vi "FPGA (Top Level).vi"() -> ()   [LabVIEW 2017]
uses:
  <vilib>/LabVIEW Targets/FPGA/cRIO/cRIO-9505/controls.llb/_nicrio_cRIO-9505_DriveStatus.ctl
  <vilib>/Platform/TimedLoop/XDataNode/timing_clust.ctl
  <vilib>/Platform/TimedLoop/XDataNode/nitl_modes.ctl
  <vilib>/Platform/TimedLoop/XDataNode/wakeup.ctl
  <vilib>/rvi/FXPMathLib/FxpSinAndCos/subVIs/nifxpmath_SinAndCos_SimConfig.ctl
  <vilib>/rvi/Emulation/niFpgaGetClockAttributes.vi
  <vilib>/rvi/Emulation/niFpgaSctlEmulationGetInTimedLoop.vi
  <vilib>/rvi/Emulation/niFpgaEmulationReportErrorSimple.vi
  <vilib>/rvi/eio/common/nirviEmuTemplateMethod_errors.vi
  <vilib>/rvi/Emulation/niFpgaEmulationIsFPGAContextNoSignature.vi
  <vilib>/rvi/DataTransferAndStorage/Container/Common/niFpgaContainerGetUniqueNameForEmu.vi
  <vilib>/rvi/Memory/Memory_Emulation/niFpgaMemoryEmulationCacheClearOnFirstRun.vi
  <vilib>/rvi/Memory/Memory_Emulation/nirvimemoryEmulationManagerCache_MakeExclusive.vi
  <vilib>/rvi/Memory/Memory_Emulation/niFpgaMemoryEmulationValidateCache.vi
  <vilib>/rvi/Memory/Memory_Emulation/nirvimemoryEmulationManagerCache_InsertValue.vi
  <vilib>/Utility/error.llb/Clear Errors.vi
  <vilib>/rvi/Memory/Memory_Emulation/nirvimemoryEmulationManagerCache_ReleaseExclusive.vi
  <vilib>/rvi/Memory/Memory_Emulation/nirvimemoryEmulationManagerCache_GetValue.vi
  <vilib>/rvi/Memory/Memory_Emulation/nirvimemoryEmulationManagerCache_SetValue.vi
  <vilib>/rvi/Emulation/niFpgaProcessEmulError.vi
  <vilib>/rvi/Emulation/niFpgaCriticalErrorInLSC.vi
  <vilib>/rvi/FXPMathLib/FxpSinAndCos/simVIs/DllFxpSinAndCosTemp_sub.vi
  <vilib>/eio/EIONode/EIONode.xnode
  <vilib>/rvi/DataTransferAndStorage/Container/XNode/niFpgaContainer.xnode
  <vilib>/rvi/DataTransferAndStorage/Register/Emulation/niFpgaRegisterEmulation.vi
  <vilib>/rvi/FXPMathLib/FxpSinAndCos/XNode/nifxpmath_SinAndCos.xnode
  <vilib>/Platform/TimedLoop/XDataNode/XDataNode.xnode
  <vilib>/Platform/TimedLoop/XDataNode/XDNodeRunTimeDep.lvlib
  <vilib>/eio/EIOMethodNode/EIOMethodNode.xnode
panel:
  out "x .or. y?":u8
  out "PWM Period (ticks)":u32
  out "Link 2 PWM Duty (Counts)":i32
  out "Link 1 PWM Duty (Counts)":i32
  in  "PWM Gen Period (ms)":u16=10
  in  "Enable Output V":bool
  in  "PWM Period Loops":i32=200
  in  "Link_1 Duty":fxp<+/-,32,0>
  in  "Link_2 Duty":fxp<+/-,32,0>
  in  "LINK1_DRIVE_ENABLED":bool
  in  "LINK2_DRIVE_ENABLED":bool
  out "LINK2_DRIVE_STATUS":T1
  out "LINK1_DRIVE_STATUS":T1
  in  "LINK1_LENGTH_MM":fxp<+,16,12>=2.0 format="%#_19g"
  in  "LINK2_LENGTH_MM":fxp<+,16,12>=2.0 format="%#_19g"
  in  "X_OFFSET_MM":fxp<+/-,33,15>
  in  "Y_OFFSET_MM":fxp<+/-,33,15>
  out "LINK2_Y_MM":fxp<+/-,34,16>
  out "LINK2_X_MM":fxp<+/-,34,16>
  out "LINK1_Y_MM":fxp<+/-,34,16>
  out "LINK1_X_MM":fxp<+/-,34,16>
  out "LINK1_ENC_POS":i32
  out "LINK2_ENC_POS":i32
  out "LINK1_POT_POS":i32
  out "LINK2_POT_POS":i32
  in  "LINK1_ENC_SCALE":fxp<+,32,0> format="%#_32g"
  in  "LINK2_ENC_SCALE":fxp<+,32,0>=0.029296900611370802 format="%#_32g"
  in  "LINK1_PWM_MAX":i16
  in  "LINK2_PWM_MAX":i16
  in  "LINK1_DEMAND_PWM":i16
  in  "LINK2_DEMAND_PWM":i16
  in  "LINK1_POT_SCALE":fxp<+/-,32,16>
  in  "LINK1_OFFSET":fxp<+/-,16,16>
  in  "LINK2_POT_SCALE":fxp<+/-,32,16>
  in  "LINK2_OFFSET":fxp<+/-,16,16>
  in  "AI_POT_LOOP_US":u16=10
  in  "ENC_DEBOUNCE_CYCLES":u16=5
  in  "LINK1_ENC_CNTS":i32
  in  "LINK2_ENC_CNTS":i32
  in  "LINK1_UPDATE_ENC":bool
  in  "LINK2_UPDATE_ENC":bool
  # "PWM at 50kHz"
  # "10MHz Loops Rate"
  # "3.3V"
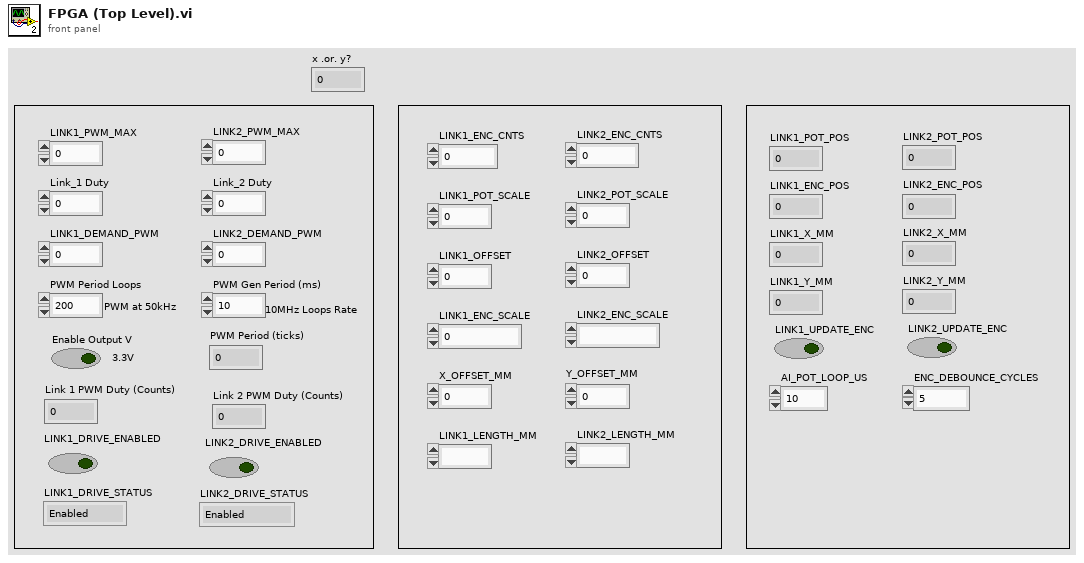
[diagram p1: front panel]
types:
  T1 = typedef "_nicrio_cRIO-9505_DriveStatus.ctl" = enum8{"Enabled", "Disabled", "Disabled by Drive Fault", "Disabled by Temp. Fault", "Disabled by E-Stop", "Unknown"}
  T2 = typedef "XDNodeRunTimeDep.lvlib/timing_clust.ctl" = cluster{"Expected End [f-1]":u64, "Actual End [f-1]":u64, "Finished Late? [f-1]":bool, "Expected End [i-1]":u64, "Actual End [i-1]":u64, "Finished Late? [i-1]":bool, "Expected Start [i]":u64, "Actual Start [i]":u64, "Expected Start [f]":u64, "Actual Start [f]":u64, "Source Name":string, "Structure Name":string, "Period":i64, "Deadline":i64, "Offset":i64, "Start":i64, "Priority":i32, "Timeout":i32, "Mode":T3, "Wakeup Reason":T4, "Error":errorcluster, "Source Type":string, "Secondary Source Type":string, "Global End Time":u64, "Global Start Time":u64, "Frame Duration":u64, "Iteration Duration":u64, "Assigned CPU":i32, "I/O Scan Engine Mode":u32}
  T3 = typedef "XDNodeRunTimeDep.lvlib/nitl_modes.ctl" = enum32{"No Change", "Process missed periods, maintain original phase", "Discard missed periods, maintain original phase", "Process missed periods, ignore original phase", "Discard missed periods, ignore original phase"}
  T4 = typedef "XDNodeRunTimeDep.lvlib/wakeup.ctl" = enum32{"Normal", "Aborted", "Asynchronous wakeup", "Timing source error", "Timed loop error", "Timeout"}
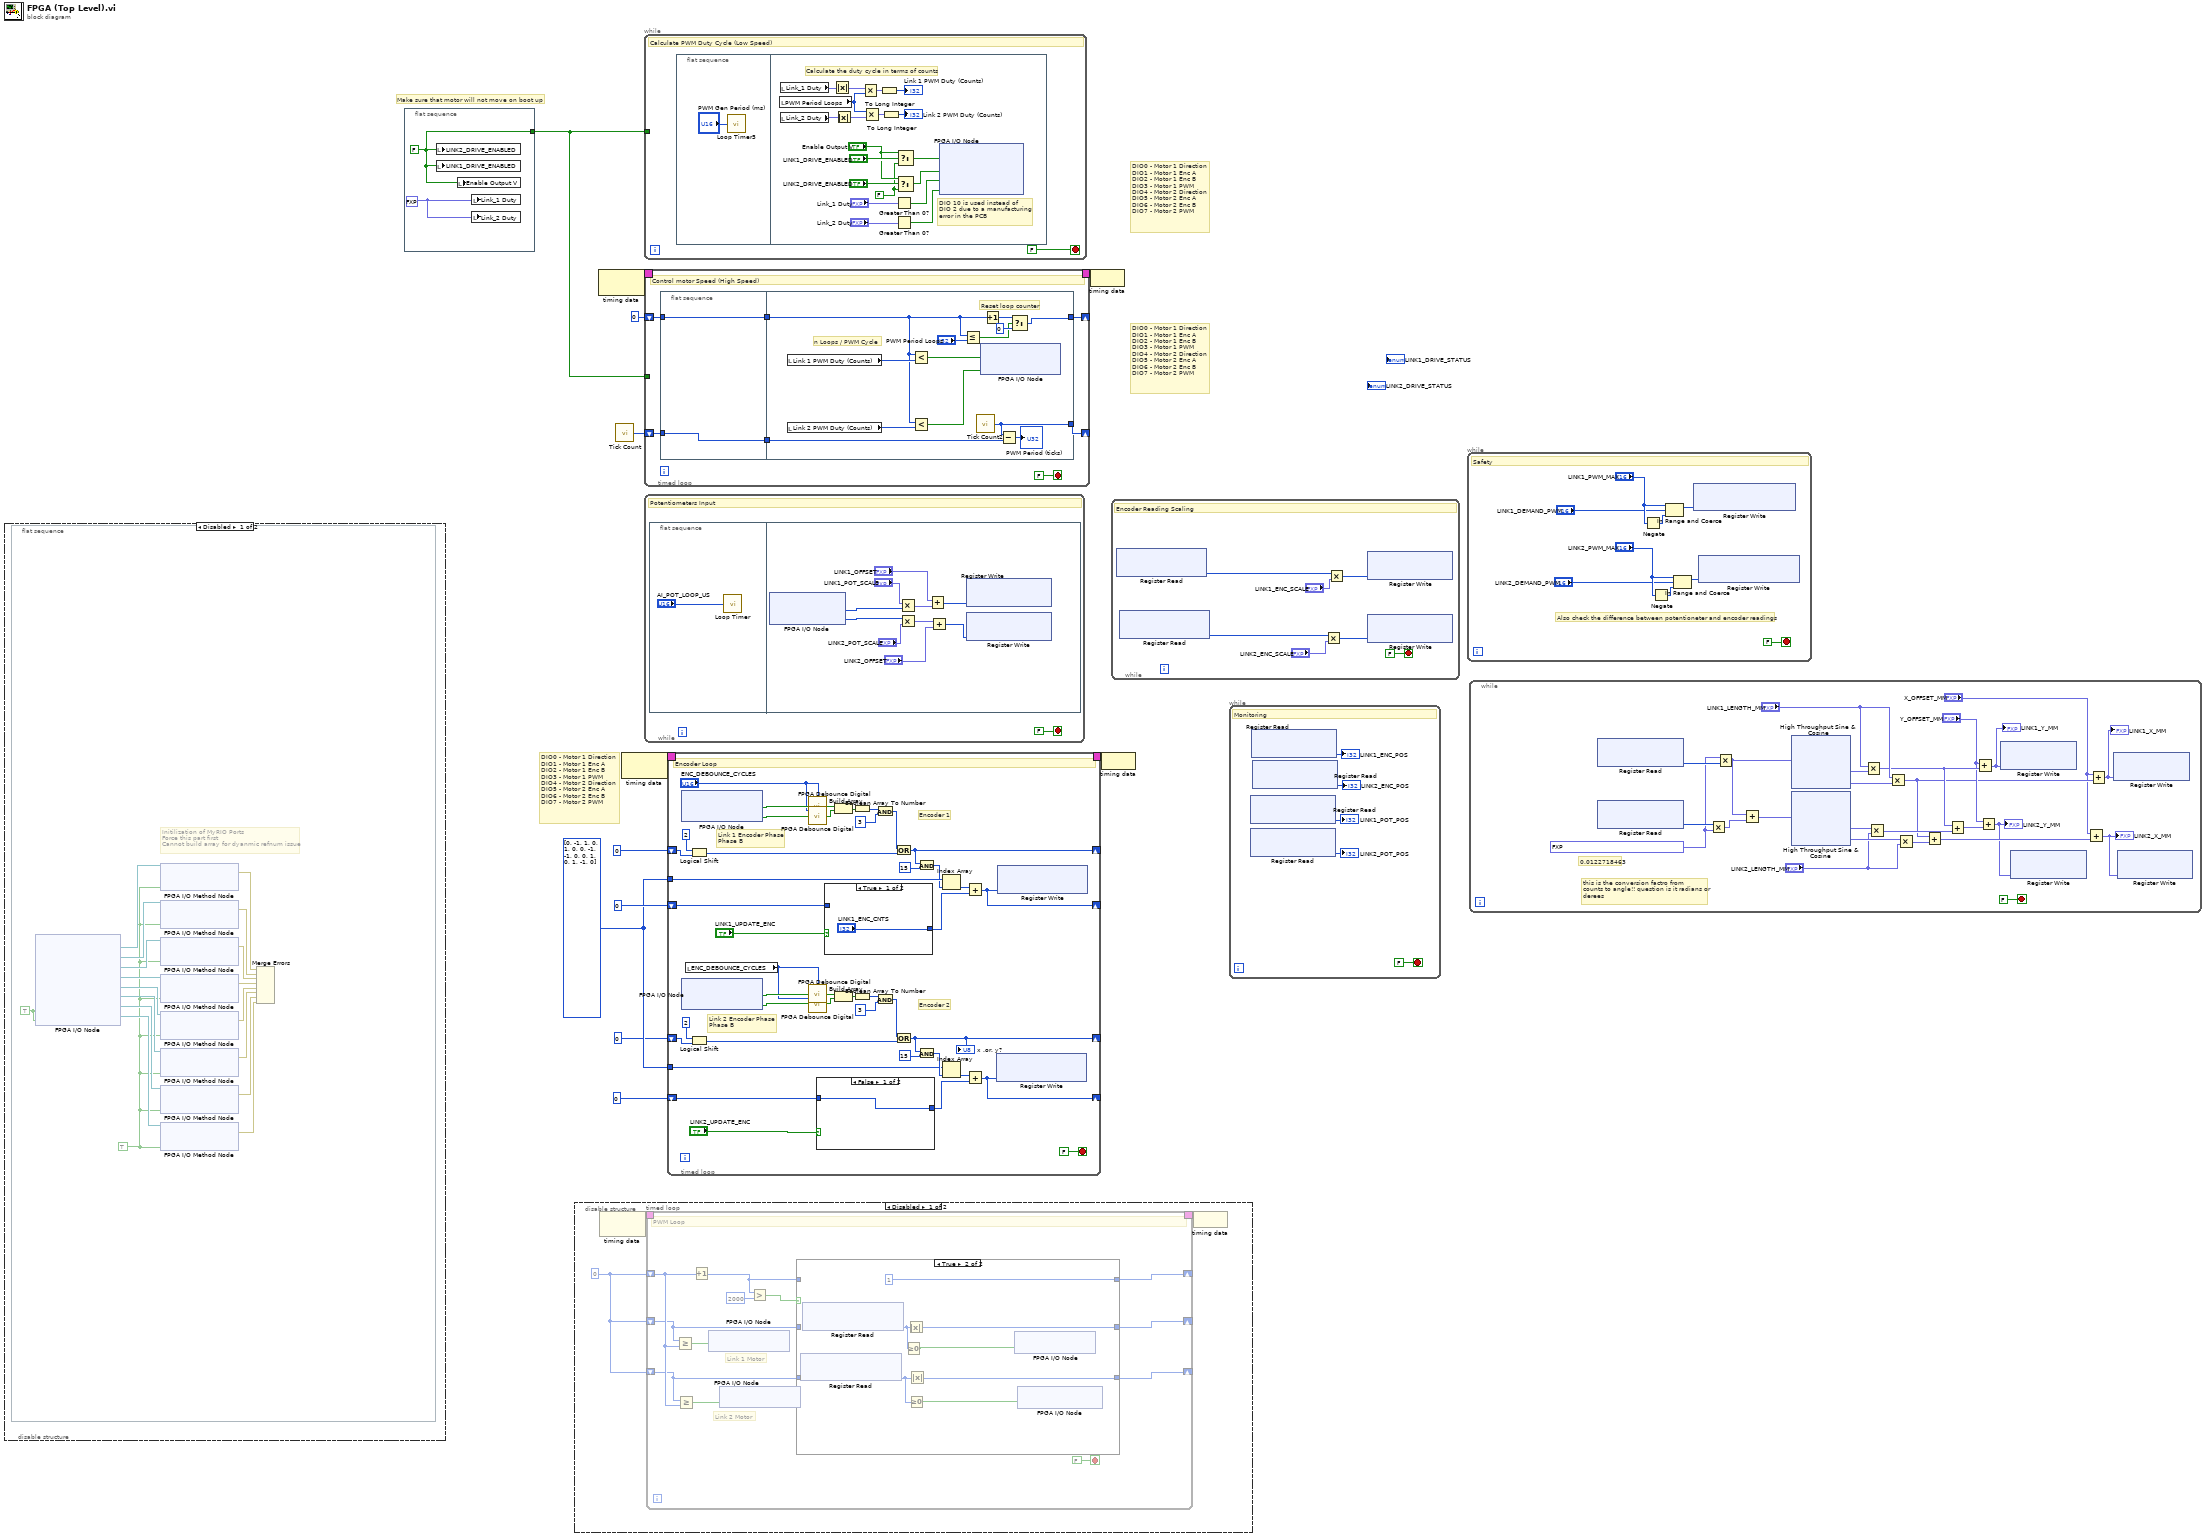
[diagram p0: block diagram]
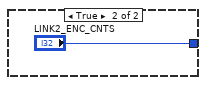
[diagram p5: hidden frame]
diagram:
  w8 = i8[] [0, -1, 1, 0, 1, 0, 0, -1, -1, 0, 0, 1, 0, 1, -1, 0]
  # "DIO0 - Motor 1 Direction \nDIO1 - Motor 1 Enc A\nDIO2 - Motor 1 Enc B\nDIO3 - Motor 1 PWM\nDIO4 - Motor 2 Direction\nDIO5 - Motor 2 Enc A\nDIO6 - Motor 2 Enc B\nDIO7 - Motor 2 PWM"
  # "DIO0 - Motor 1 Direction \nDIO1 - Motor 1 Enc A\nDIO2 - Motor 1 Enc B\nDIO3 - Motor 1 PWM\nDIO4 - Motor 2 Direction\nDIO5 - Motor 2 Enc A\nDIO6 - Motor 2 Enc B\nDIO7 - Motor 2 PWM"
  # "DIO0 - Motor 1 Direction \nDIO1 - Motor 1 Enc A\nDIO2 - Motor 1 Enc B\nDIO3 - Motor 1 PWM\nDIO4 - Motor 2 Direction\nDIO5 - Motor 2 Enc A\nDIO6 - Motor 2 Enc B\nDIO7 - Motor 2 PWM"
  # "Make sure that motor will not move on boot up"
  n1 = disable-structure shown="Disabled" {
    frame Disabled {
      n2 = flat-sequence {
        frame #0 {
          w21 = TRUE ("Link 2 Encoder Phase B")
          w30 = TRUE ("Link 2 Encoder Phase B")
          # "Initilization of MyRIO Ports\nForce this part first \nCannot build array for dyanmic refnum issue"
          n3 = xnode "FPGA I/O Node"("ConnectorA/DIO5"=w30, "ConnectorA/DIO10"=w30) -> ("FPGA I/O Out"=w29:refnum<k21>, "FPGA I/O Out"=w28:refnum<k21>, "FPGA I/O Out"=w27:refnum<k21>, "FPGA I/O Out"=w26:refnum<k21>, "FPGA I/O Out"=w25:refnum<k21>, "FPGA I/O Out"=w24:refnum<k21>, "FPGA I/O Out"=w23:refnum<k21>, "FPGA I/O Out"=w22:refnum<k21>)  [unwired: 8 in, 6 out]
          n4 = xnode "FPGA I/O Method Node"("FPGA I/O In"=w29, "Enable"=w21) -> ("error out"=w20:errorcluster)  [unwired: 1 in, 1 out]
          n5 = xnode "FPGA I/O Method Node"("FPGA I/O In"=w28, "Enable"=w21) -> ("error out"=w19:errorcluster)  [unwired: 1 in, 1 out]
          n6 = xnode "FPGA I/O Method Node"("FPGA I/O In"=w27, "Enable"=w21) -> ("error out"=w18:errorcluster)  [unwired: 1 in, 1 out]
          n7 = xnode "FPGA I/O Method Node"("FPGA I/O In"=w26, "Enable"=w21) -> ("error out"=w17:errorcluster)  [unwired: 1 in, 1 out]
          n8 = xnode "FPGA I/O Method Node"("FPGA I/O In"=w25, "Enable"=w21) -> ("error out"=w16:errorcluster)  [unwired: 1 in, 1 out]
          n9 = xnode "FPGA I/O Method Node"("FPGA I/O In"=w24, "Enable"=w21) -> ("error out"=w15:errorcluster)  [unwired: 1 in, 1 out]
          n10 = xnode "FPGA I/O Method Node"("FPGA I/O In"=w23, "Enable"=w21) -> ("error out"=w14:errorcluster)  [unwired: 1 in, 1 out]
          n11 = xnode "FPGA I/O Method Node"("FPGA I/O In"=w22, "Enable"=w21) -> ("error out"=w13:errorcluster)  [unwired: 1 in, 1 out]
          n12 = Merge Errors(w20, w19, w18, w17, w16, w15, w14, w13) -> ()  [unwired: 1 out]
        }
      }
    }
    frame Enabled {
    }
  }
  n13 = flat-sequence {
    tunnel: [w31] -> w1
    frame #0 {
      w32 = fxp<+/-,32,0> 0.0 ("Link_1 Duty")
      w31 = FALSE ("LINK2_DRIVE_ENABLED")
      n14 = local write "LINK2_DRIVE_ENABLED"(w31) -> ()
      n15 = local write "LINK1_DRIVE_ENABLED"(w31) -> ()
      n16 = local write "Enable Output V"(w31) -> ()
      n17 = local write "Link_1 Duty"(w32) -> ()
      n18 = local write "Link_2 Duty"(w32) -> ()
    }
  }
  n19 = disable-structure shown="Disabled" {
    frame Disabled {
      w33 = i16 0 ("Motor 1 PWM Duty Cycle")
      n20 = node-c288() -> (w35:T2)  [unwired: 1 in]
      n21 = timed-loop {
        timing: w35 -> [_]
        timing-out: [_] -> w34
        shift-right: [w46] -> _
        shift-left: w33 -> [w45]
        shift-right: [w44] -> _
        shift-left: w33 -> [w42]
        shift-right: [w43] -> _
        shift-left: w33 -> [w41]
        stop <- FALSE stop-if-true
        # "Link 2 Motor"
        # "Link 1 Motor"
        # "PWM Loop"
        n22 = Greater Or Equal?(x=w42, y=w45) -> (x >= y?=w37:bool)
        n23 = Greater Or Equal?(x=w41, y=w45) -> (x >= y?=w36:bool)
        n24 = Increment(x=w45) -> (x+1=w39:i16)
        n25 = xnode "FPGA I/O Node"("ConnectorA/DIO8"=w37) -> ()  [unwired: 1 in, 1 out]
        n26 = xnode "FPGA I/O Node"("ConnectorA/DIO9"=w36) -> ()  [unwired: 1 in, 1 out]
        n27 = Greater?(x=w39, y=i16 2000) -> (0:w40:bool)
        n28 = case shown="True" w40 {
          tunnel: w39 -> [w50 _]
          tunnel: [w50 i16 1 ("Motor 1 PWM Duty Cycle")] -> w46
          tunnel: [w49 w56] -> w44
          tunnel: [w48 w55] -> w43
          tunnel: w42 -> [w49 _]
          tunnel: w41 -> [w48 _]
          frame False {
          }
          frame True {
            n29 = xnode ("Register Read")() -> ("Data"=w53:i16)  [unwired: 1 in, 1 out]
            n30 = xnode ("Register Read")() -> ("Data"=w54:i16)  [unwired: 1 in, 1 out]
            n31 = Greater Or Equal To 0?(x=w54) -> (x >= 0?=w51:bool)
            n32 = Absolute Value(x=w54) -> (abs(x)=w56:i16)
            n33 = Greater Or Equal To 0?(x=w53) -> (x >= 0?=w52:bool)
            n34 = Absolute Value(x=w53) -> (abs(x)=w55:i16)
            n35 = xnode "FPGA I/O Node"("ConnectorA/DIO6"=w51) -> ()  [unwired: 1 in, 1 out]
            n36 = xnode "FPGA I/O Node"("ConnectorA/DIO10"=w52) -> ()  [unwired: 1 in, 1 out]
          }
        }
      }
      n37 = node-c288(w34) -> ()
    }
    frame Enabled {
    }
  }
  n38 = node-c288() -> (w4:T2)  [unwired: 1 in]
  n39 = call "Tick Count"() -> ("Tick Count(Ticks)"=w5:u32)
  n40 = node-c288() -> (w12:T2)  [unwired: 1 in]
  n41 = while {
    tunnel: w1 -> [_]
    stop <- FALSE stop-if-true
    # "Calculate PWM Duty Cycle (Low Speed)"
    n42 = flat-sequence {
      frame #0 {
        n43 = call "Loop Timer3"("Count(mSec)"="PWM Gen Period (ms)") -> ()  [unwired: 1 out]
      }
      frame #1 {
        w70 = FALSE
        # "DIO 10 is used instead of \nDIO 2 due to a manufacturing \nerror in the PCB"
        # "Calculate the duty cycle in terms of counts"
        n44 = local read "PWM Period Loops"() -> (w74:i32)
        n45 = local read "Link_1 Duty"() -> (w79:fxp<+/-,32,0>)
        n46 = local read "Link_2 Duty"() -> (w75:fxp<+/-,32,0>)
        n47 = Absolute Value(x=w79) -> (abs(x)=w80:fxp<+,32,0>)
        n48 = Absolute Value(x=w75) -> (abs(x)=w76:fxp<+,32,0>)
        n49 = Multiply(x=w80, y=w74) -> (x*y=w81:fxp<+/-,63,31>)
        n50 = Multiply(x=w74, y=w76) -> (x*y=w78:fxp<+/-,63,31>)
        n51 = To Long Integer(number=w81) -> (32bit integer=→"Link 1 PWM Duty (Counts)":i32)
        n52 = To Long Integer(number=w78) -> (32bit integer=→"Link 2 PWM Duty (Counts)":i32)
        n53 = Greater Than 0?(x="Link_1 Duty") -> (x > 0?=w65:bool)
        n54 = Greater Than 0?(x="Link_2 Duty") -> (x > 0?=w64:bool)
        n55 = Select(t="Enable Output V", s="LINK1_DRIVE_ENABLED", f=w70) -> (s? t:f=w69:bool)
        n56 = Select(t="Enable Output V", s="LINK2_DRIVE_ENABLED", f=w70) -> (s? t:f=w68:bool)
        n57 = xnode "FPGA I/O Node"("ConnectorA/DIO10"=w69, "ConnectorA/DIO7"=w68, "ConnectorA/DIO0"=w65, "ConnectorA/DIO5"=w64) -> ()  [unwired: 4 in, 4 out]
      }
    }
  }
  n58 = timed-loop {
    shift-right: [w88] -> _
    shift-left: w5 -> [w87]
    timing: w4 -> [_]
    timing-out: [_] -> w3
    shift-right: [w85] -> _
    shift-left: i16 0 -> [w84]
    tunnel: w1 -> [_]
    stop <- FALSE stop-if-true
    # "Control motor Speed (High Speed)"
    n59 = flat-sequence {
      tunnel: w87 -> [w91]
      tunnel: [w91] -> w86
      tunnel: w84 -> [w90]
      tunnel: [w90] -> w83
      tunnel: [w100] -> w88
      tunnel: w86 -> [w99]
      tunnel: [w96] -> w85
      tunnel: w83 -> [w93]
      frame #0 {
      }
      frame #1 {
        # "Reset loop counter"
        # "n Loops / PWM Cycle"
        n60 = local read "Link 1 PWM Duty (Counts)"() -> (w102:i32)
        n61 = local read "Link 2 PWM Duty (Counts)"() -> (w101:i32)
        n62 = Less?(x=w93, y=w102) -> (x < y?=w104:bool)
        n63 = Less?(x=w93, y=w101) -> (x < y?=w103:bool)
        n64 = Less Or Equal?(x=w93, y="PWM Period Loops") -> (x <= y?=w92:bool)
        n65 = call "Tick Count2"() -> ("Tick Count(Ticks)"=w100:u32)
        n66 = xnode "FPGA I/O Node"("ConnectorA/DIO1"=w104, "ConnectorA/DIO6"=w103) -> ()  [unwired: 2 in, 2 out]
        n67 = Increment(x=w93) -> (x+1=w97:i16)
        n68 = Subtract(x=w100, y=w99) -> (x-y=→"PWM Period (ticks)":u32)
        n69 = Select(t=w97, s=w92, f=i16 0) -> (s? t:f=w96:i16)
      }
    }
  }
  n70 = while {
    stop <- FALSE stop-if-true
    # "Potentiometers Input"
    n71 = flat-sequence {
      frame #0 {
        n72 = call "Loop Timer"("Count(uSec)"="AI_POT_LOOP_US") -> ()  [unwired: 1 out]
      }
      frame #1 {
        n73 = xnode "FPGA I/O Node"() -> ("ConnectorA/AI1"=w110:u16, "ConnectorA/AI2"=w109:u16)  [unwired: 2 in, 2 out]
        n74 = Multiply(x="LINK1_POT_SCALE", y=w110) -> (x*y=w117:fxp<+/-,48,32>)
        n75 = Multiply(x=w109, y="LINK2_POT_SCALE") -> (x*y=w113:fxp<+/-,48,32>)
        n76 = Add(x="LINK1_OFFSET", y=w117) -> (x+y=w111:i32)
        n77 = Add(x=w113, y="LINK2_OFFSET") -> (x+y=w112:i32)
        n78 = xnode ("Register Write")("Data"=w111) -> ()  [unwired: 1 in, 1 out]
        n79 = xnode ("Register Write")("Data"=w112) -> ()  [unwired: 1 in, 1 out]
      }
    }
  }
  n80 = timed-loop {
    timing: w12 -> [_]
    timing-out: [_] -> w11
    tunnel: w8 -> [w158]
    shift-right: [w151] -> _
    shift-left: u8 0 -> [w160]
    shift-right: [w122] -> _
    shift-left: 0 -> [w143]
    tunnel: w8 -> [w127]
    shift-right: [w125] -> _
    shift-left: u8 0 -> [w126]
    shift-right: [w121] -> _
    shift-left: 0 -> [w119]
    stop <- FALSE stop-if-true
    # "Link 2 Encoder Phase \nPhase B"
    # "Link 1 Encoder Phase \nPhase B"
    # "Encoder 2"
    # "Encoder 1"
    # "Encoder Loop"
    n81 = xnode "FPGA I/O Node"() -> ("ConnectorA/DIO4"=w149:bool, "ConnectorA/DIO3"=w148:bool)  [unwired: 2 in, 2 out]
    n82 = xnode "FPGA I/O Node"() -> ("ConnectorA/DIO9"=w133:bool, "ConnectorA/DIO8"=w132:bool)  [unwired: 2 in, 2 out]
    n83 = local read "ENC_DEBOUNCE_CYCLES"() -> (w124:u16)
    n84 = Logical Shift(y=i16 2, x=w160) -> (x << y=w153:u8)
    n85 = Logical Shift(y=i16 2, x=w126) -> (x << y=w136:u8)
    n86 = call "FPGA Debounce Digital.vi"("Input Signal"=w149, "Cycles to Filter"="ENC_DEBOUNCE_CYCLES") -> ("Output Filtered Signal"=w147:bool)
    n87 = call "FPGA Debounce Digital.vi"("Input Signal"=w148, "Cycles to Filter"="ENC_DEBOUNCE_CYCLES") -> ("Output Filtered Signal"=w146:bool)
    n88 = call "FPGA Debounce Digital.vi"("Input Signal"=w133, "Cycles to Filter"=w124) -> ("Output Filtered Signal"=w131:bool)
    n89 = call "FPGA Debounce Digital.vi"("Input Signal"=w132, "Cycles to Filter"=w124) -> ("Output Filtered Signal"=w130:bool)
    n90 = case shown="False" "LINK2_UPDATE_ENC" {
      tunnel: w119 -> [w162 _]
      tunnel: [w162 "LINK2_ENC_CNTS"] -> w128
      frame False {
      }
      frame True {
      }
    }
    n91 = case shown="True" "LINK1_UPDATE_ENC" {
      tunnel: w143 -> [_ w165]
      tunnel: ["LINK1_ENC_CNTS" w165] -> w142
      frame True {
      }
      frame False {
      }
    }
    n92 = Build Array(w147, w146) -> (w145:bool[])
    n93 = Build Array(w131, w130) -> (w129:bool[])
    n94 = Boolean Array To Number(Boolean array=w145) -> (number=w156:u8)
    n95 = Boolean Array To Number(Boolean array=w129) -> (number=w139:u8)
    n96 = And(x=w156, y=u8 3) -> (x .and. y?=w154:u8)
    n97 = And(x=w139, y=u8 3) -> (x .and. y?=w137:u8)
    n98 = Or(x=w154, y=w153) -> (x .or. y?=w151:u8)
    n99 = Or(x=w137, y=w136) -> (x .or. y?=w125:u8)
    "x .or. y?" <- w125
    n100 = And(x=w151, y=u8 15) -> (x .and. y?=w152:u8)
    n101 = And(x=w125, y=u8 15) -> (x .and. y?=w135:u8)
    n102 = Index Array(array=w158, index=w152) -> (element=w150:i8)
    n103 = Index Array(array=w127, index=w135) -> (element=w134:i8)
    n104 = Add(x=w150, y=w142) -> (x+y=w122:i32)
    n105 = Add(x=w134, y=w128) -> (x+y=w121:i32)
    n106 = xnode ("Register Write")("Data"=w121) -> ()  [unwired: 1 in, 1 out]
    n107 = xnode ("Register Write")("Data"=w122) -> ()  [unwired: 1 in, 1 out]
  }
  n108 = node-c288(w3) -> ()
  n109 = node-c288(w11) -> ()
  n110 = while {
    stop <- FALSE stop-if-true
    # "Encoder Reading Scaling"
    n111 = xnode ("Register Read")() -> ("Data"=w172:i32)  [unwired: 1 in, 1 out]
    n112 = xnode ("Register Read")() -> ("Data"=w173:i32)  [unwired: 1 in, 1 out]
    n113 = Multiply(x=w173, y="LINK2_ENC_SCALE") -> (x*y=w170:i32)
    n114 = Multiply(x=w172, y="LINK1_ENC_SCALE") -> (x*y=w171:i32)
    n115 = xnode ("Register Write")("Data"=w171) -> ()  [unwired: 1 in, 1 out]
    n116 = xnode ("Register Write")("Data"=w170) -> ()  [unwired: 1 in, 1 out]
  }
  n117 = while {
    stop <- FALSE stop-if-true
    # "Monitoring"
    n118 = xnode ("Register Read")() -> ("Data"=→"LINK1_POT_POS":i32)  [unwired: 1 in, 1 out]
    n119 = xnode ("Register Read")() -> ("Data"=→"LINK2_POT_POS":i16)  [unwired: 1 in, 1 out]
    n120 = xnode ("Register Read")() -> ("Data"=→"LINK1_ENC_POS":i32)  [unwired: 1 in, 1 out]
    n121 = xnode ("Register Read")() -> ("Data"=→"LINK2_ENC_POS":i32)  [unwired: 1 in, 1 out]
  }
  n122 = while {
    stop <- FALSE stop-if-true
    # "Also check the difference between potentioneter and encoder readings"
    # "Safety"
    n123 = Negate(x="LINK1_PWM_MAX") -> (-x=w186:i16)
    n124 = Negate(x="LINK2_PWM_MAX") -> (-x=w184:i16)
    n125 = In Range and Coerce(upper limit="LINK1_PWM_MAX", x="LINK1_DEMAND_PWM", lower limit=w186) -> (coerced(x)=w187:i16)  [unwired: 1 out]
    n126 = In Range and Coerce(upper limit="LINK2_PWM_MAX", x="LINK2_DEMAND_PWM", lower limit=w184) -> (coerced(x)=w183:i16)  [unwired: 1 out]
    n127 = xnode ("Register Write")("Data"=w187) -> ()  [unwired: 1 in, 1 out]
    n128 = xnode ("Register Write")("Data"=w183) -> ()  [unwired: 1 in, 1 out]
  }
  n129 = while {
    stop <- FALSE stop-if-true
    w189 = fxp<+,31,-8> 5.555555617320351e-05
    # "0.0122718463"
    # "this is the conversion factro from \ncounts to angle!! question is it radians or\nderees"
    n130 = xnode ("Register Read")() -> ("Data"=w195:i32)  [unwired: 1 in, 1 out]
    n131 = xnode ("Register Read")() -> ("Data"=w212:i32)  [unwired: 1 in, 1 out]
    n132 = Multiply(x=w212, y=w189) -> (x*y=w211:fxp<+/-,63,24>)
    n133 = Multiply(x=w189, y=w195) -> (x*y=w194:fxp<+/-,63,24>)
    n134 = Add(x=w194, y=w211) -> (x+y=w210:fxp<+/-,64,25>)
    n135 = xnode "High Throughput Sine & Cosine"("x (pi)"=w194) -> ("sin(x)"=w209:fxp<+/-,16,2>, "cos(x)"=w208:fxp<+/-,16,2>)
    n136 = xnode "High Throughput Sine & Cosine"("x (pi)"=w210) -> ("sin(x)"=w206:fxp<+/-,16,2>, "cos(x)"=w205:fxp<+/-,16,2>)
    n137 = Multiply(x="LINK1_LENGTH_MM", y=w209) -> (x*y=w201:fxp<+/-,32,14>)
    n138 = Multiply(x=w206, y="LINK2_LENGTH_MM") -> (x*y=w202:fxp<+/-,32,14>)
    n139 = Multiply(x="LINK1_LENGTH_MM", y=w208) -> (x*y=w198:fxp<+/-,32,14>)
    n140 = Multiply(x=w205, y="LINK2_LENGTH_MM") -> (x*y=w203:fxp<+/-,32,14>)
    n141 = Add(x=w198, y=w203) -> (x+y=w197:fxp<+/-,33,15>)
    n142 = Add(x=w201, y=w202) -> (x+y=w200:fxp<+/-,33,15>)
    n143 = Add(x="Y_OFFSET_MM", y=w201) -> (x+y=w191:fxp<+/-,34,16>)
    "LINK1_Y_MM" <- w191
    n144 = Add(x="Y_OFFSET_MM", y=w200) -> (x+y=w193:fxp<+/-,34,16>)
    "LINK2_Y_MM" <- w193
    n145 = xnode ("Register Write")("Data"=w191) -> ()  [unwired: 1 in, 1 out]
    n146 = xnode ("Register Write")("Data"=w193) -> ()  [unwired: 1 in, 1 out]
    n147 = Add(x="X_OFFSET_MM", y=w197) -> (x+y=w192:fxp<+/-,34,16>)
    "LINK2_X_MM" <- w192
    n148 = Add(x="X_OFFSET_MM", y=w198) -> (x+y=w190:fxp<+/-,34,16>)
    "LINK1_X_MM" <- w190
    n149 = xnode ("Register Write")("Data"=w190) -> ()  [unwired: 1 in, 1 out]
    n150 = xnode ("Register Write")("Data"=w192) -> ()  [unwired: 1 in, 1 out]
  }
